vi "KNN.vi"(11 "SD from Arduino":dbl=2.0 format="%#_13g") -> (3 "element":dbl)   [LabVIEW 2021]
uses:
  b18fc042-107d-9545-9343-fca6f8f5a483.vi
  9f81a91f-1fb0-674e-877a-d2309b603bf6.vi
  c0752967-5801-0547-bad4-bbc4b5936bff.vi
  af8ebcad-f16b-5448-b96b-68c09163bebe.vi
  284cf464-ac97-1240-b04e-2dce3663e608.vi
  <vilib>/Array/Sort 2D Array - Pop Stack.vi
  <vilib>/Array/Sort 2D Array - Push Stack.vi
  284cf464-ac97-1240-b04e-2dce3663e608.vi/269d4b3b-47f5-49e3-8884-44851e4dd9d5.vi
  284cf464-ac97-1240-b04e-2dce3663e608.vi/6d99389c-673d-4efb-bf33-19b32bcf4cf8.vi
  <vilib>/Utility/file.llb/Read Delimited Spreadsheet (DBL).vi
  <vilib>/Comparison/Less/Less Functor/Less Functor.lvclass
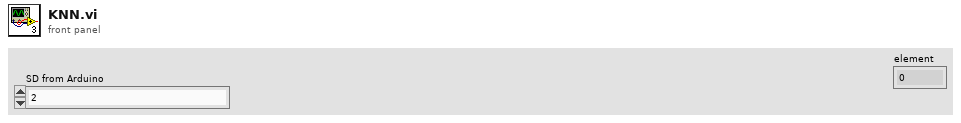
[diagram p1: front panel]
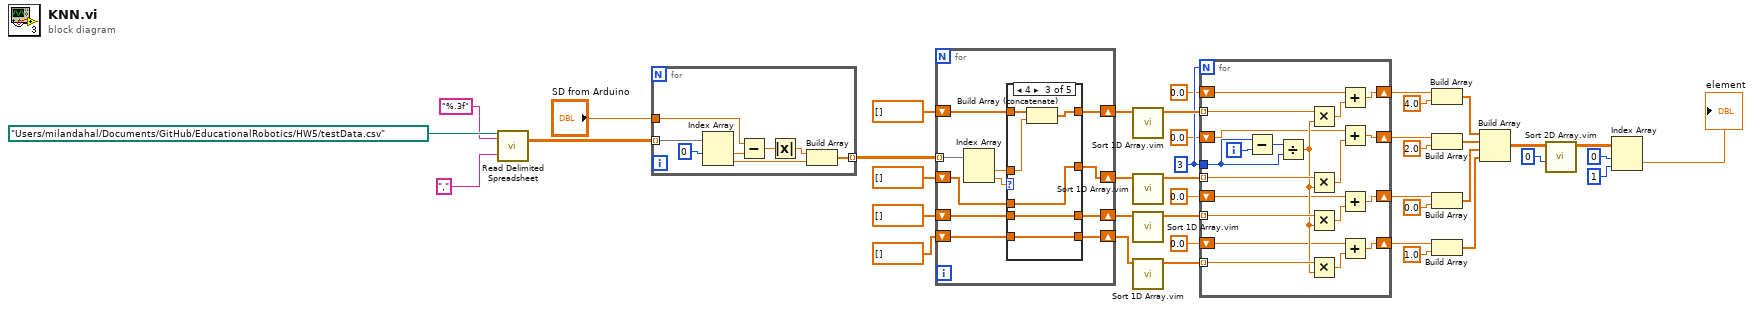
[diagram p0: block diagram]
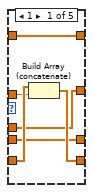
[diagram p2: hidden frame]
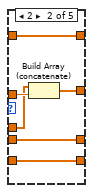
[diagram p3: hidden frame]
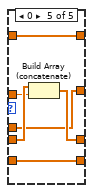
[diagram p5: hidden frame]
diagram:
  w23 = 3
  n1 = call-poly <vilib>:"Read Delimited Spreadsheet.vi"("file path (dialog if empty)"=path "/Users/milandahal/Documents/GitHub/EducationalRobotics/HW5/testData.csv", "format (%.3f)"="%.3f", "delimiter (\\t)"="," ("delimiter (\\t)")) -> ("all rows"=w34:dbl[][])  [unwired: 7 in, 5 out]
  n2 = for {
    tunnel: w34 -> [w46] mode=indexing
    tunnel: "SD from Arduino" -> [w49]
    tunnel: [w42] -> w32 mode=indexing
    n3 = Index Array(array=w46, index #1=0 ("index")) -> (element #1=w44:dbl, element #2=w43:dbl)  [unwired: 1 in]
    n4 = Subtract(x=w49, y=w44) -> (x-y=w48:dbl)
    n5 = Absolute Value(x=w48) -> (abs(x)=w47:dbl)
    n6 = Build Array(w47, w43) -> (w42:dbl[])
  }
  n7 = for {
    tunnel: w32 -> [w60] mode=indexing
    shift-right: [w50] -> w31
    shift-left: dbl[] [] -> [w57]
    shift-right: [w55] -> w30
    shift-left: dbl[] [] -> [w56]
    shift-right: [w53] -> w28
    shift-left: dbl[] [] -> [w54]
    shift-right: [w51] -> w29
    shift-left: dbl[] [] -> [w52]
    n8 = Index Array(array=w60) -> (element #1=w58:dbl, element #2=w59:dbl)  [unwired: 2 in]
    n9 = case shown="4" w59 {
      tunnel: w58 -> [w65 w72 w77 _ w87]
      tunnel: w57 -> [w63 w70 w75 w82 w88]
      tunnel: w56 -> [w66 w69 w74 w81 w85]
      tunnel: [w64 w69 w74 w81 w85] -> w55
      tunnel: w54 -> [w62 w68 w73 w80 w84]
      tunnel: [w62 w71 w73 w80 w84] -> w53
      tunnel: w52 -> [w61 w67 w78 w79 w83]
      tunnel: [w61 w67 w76 w79 w83] -> w51
      tunnel: [w63 w70 w75 w82 w86] -> w50
      frame 1 {
        n10 = Build Array (concatenate)(w66, w65) -> (w64:dbl[])
      }
      frame 2 {
        n11 = Build Array (concatenate)(w68, w72) -> (w71:dbl[])
      }
      frame 4 {
        n12 = Build Array (concatenate)(w78, w77) -> (w76:dbl[])
      }
      frame Default {
      }
      frame 0 {
        n13 = Build Array (concatenate)(w88, w87) -> (w86:dbl[])
      }
    }
  }
  n14 = call "Sort 1D Array.vim"("unsorted array"=w29) -> ("sorted array"=w25:dbl[])  [unwired: 10 in]
  n15 = call "Sort 1D Array.vim"("unsorted array"=w28) -> ("sorted array"=w24:dbl[])  [unwired: 10 in]
  n16 = call "Sort 1D Array.vim"("unsorted array"=w31) -> ("sorted array"=w27:dbl[])  [unwired: 10 in]
  n17 = call "Sort 1D Array.vim"("unsorted array"=w30) -> ("sorted array"=w26:dbl[])  [unwired: 10 in]
  n18 = for {
    N: w23 -> [_]
    tunnel: w27 -> [w105] mode=indexing
    tunnel: w26 -> [w104] mode=indexing
    tunnel: w25 -> [w103] mode=indexing
    tunnel: w24 -> [w102] mode=indexing
    tunnel: w23 -> [w106]
    shift-right: [w92] -> w18
    shift-left: 0.0 -> [w94]
    shift-right: [w89] -> w16
    shift-left: 0.0 -> [w91]
    shift-right: [w95] -> w12
    shift-left: 0.0 -> [w96]
    shift-right: [w97] -> w14
    shift-left: 0.0 -> [w98]
    i -> [w108]
    n19 = Subtract(x=w106, y=w108) -> (x-y=w107:i32)
    n20 = Divide(x=w107, y=w106) -> (x/y=w101:dbl)
    n21 = Multiply(x=w103, y=w101) -> (x*y=w93:dbl)
    n22 = Multiply(x=w102, y=w101) -> (x*y=w90:dbl)
    n23 = Multiply(x=w105, y=w101) -> (x*y=w100:dbl)
    n24 = Multiply(x=w104, y=w101) -> (x*y=w99:dbl)
    n25 = Add(x=w94, y=w93) -> (x+y=w92:dbl)
    n26 = Add(x=w91, y=w90) -> (x+y=w89:dbl)
    n27 = Add(x=w98, y=w100) -> (x+y=w97:dbl)
    n28 = Add(x=w96, y=w99) -> (x+y=w95:dbl)
  }
  n29 = Build Array(w18, 4.0 ("element")) -> (w10:dbl[])
  n30 = Build Array(w16, 2.0 ("element")) -> (w9:dbl[])
  n31 = Build Array(w14, 0.0 ("element")) -> (w8:dbl[])
  n32 = Build Array(w12, 1.0 ("element")) -> (w7:dbl[])
  n33 = Build Array(w10, w9, w8, w7) -> (w6:dbl[][])
  n34 = call "Sort 2D Array.vim"("index"=0, "2D array"=w6) -> ("sorted 2D array"=w4:dbl[][])  [unwired: 8 in, 1 out]
  n35 = Index Array(array=w4, index (row)=0, index (col)=1 ("disabled index (col)")) -> (element=→"element":dbl)
